vi "Read Download Path.vi"() -> (0 "error out":errorcluster, 3 "Download Path":path)   [LabVIEW 2024, in "Word Search Scorer.lvlib"]
uses:
  Word Search Scorer.lvlib
  <vilib>/Utility/config.llb/NI_LVConfig.lvlib
  <vilib>/Utility/config.llb/Read Key (Path).vi
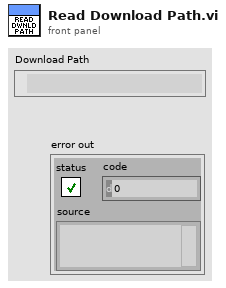
[diagram p1: front panel]
types:
  T1 = typedef "NI_LVConfig.lvlib/Config Data RefNum.ctl" = refnum<k1>
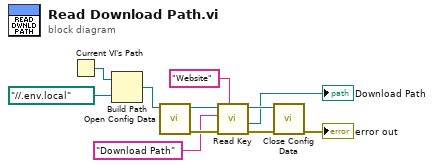
[diagram p0: block diagram]
diagram:
  n1 = Current VI's Path() -> (path=w11:path)
  n2 = Build Path(base path=w11, name or relative path=path "../../.env.local") -> (appended path=w9:path)
  n3 = call <vilib>:"Open Config Data.vi"("configuration file path"=w9) -> ("error out"=w8:errorcluster, "refnum"=w7:T1)  [unwired: 8 in, 1 out]
  n4 = call-poly <vilib>:"Read Key.vi"("section"="Website", "error in (no error)"=w8, "key"="Download Path", "refnum"=w7) -> ("error out"=w5:errorcluster, "value"=→"Download Path":path, "refnum out"=w4:T1)  [unwired: 4 in, 1 out]
  n5 = call <vilib>:"Close Config Data.vi"("error in (no error)"=w5, "refnum"=w4) -> ("error out"=→"error out":errorcluster)  [unwired: 8 in, 1 out]
